vi "Read Stats.vi"(8 "error in (no error)":errorcluster, 11 "System Health Module in":refnum<class "System Health Module.lvclass">) -> (0 "error out":errorcluster, 3 "System Health Module out":refnum<class "System Health Module.lvclass">)   [LabVIEW 2020, in "Volatus.lvlib" / "System Health Module.lvclass"]
uses:
  System Health Module.lvclass
  System Health Module.lvclass/System Health Module.ctl
  System SAL/System SAL.lvclass
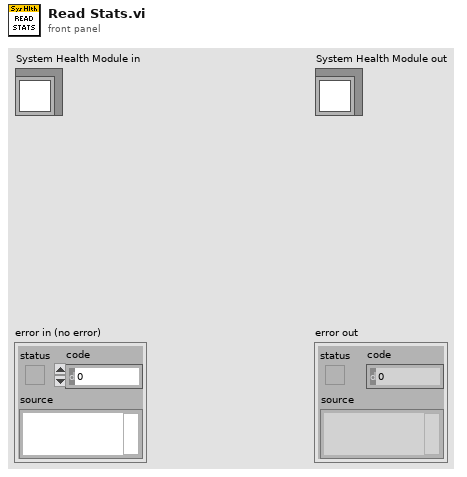
[diagram p1: front panel]
types:
  T1 = typedef "Volatus.lvlib/System Health Module.lvclass/Drive Info.ctl" = cluster{"Config":T2, "Capacity GB":dbl, "Used GB":dbl, "Last Warning":dbl, "Last Error":dbl}
  T2 = typedef "Volatus.lvlib/System Health Module.lvclass/Drive Config.ctl" = cluster{"Path":path, "Warning GB":dbl, "Error GB":dbl}
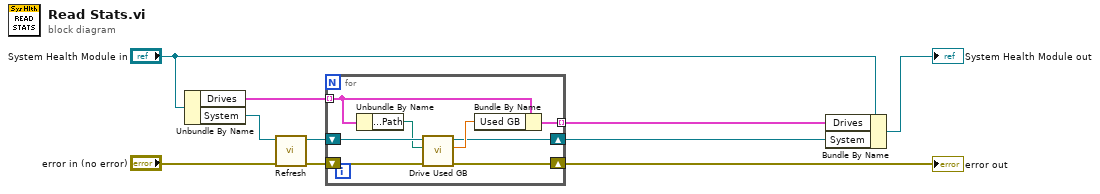
[diagram p0: block diagram]
diagram:
  n1 = Unbundle By Name("System Health Module in") -> ("Drives"=w4:T1[], "System"=w8:refnum<class "System SAL.lvclass">)
  n2 = call-dynamic "Refresh.vi"("error in (no error)"="error in (no error)", "System SAL in"=w8) -> ("error out"=w6:errorcluster, "System SAL out"=w7:refnum<class "System SAL.lvclass">)  [unwired: 8 in]
  n3 = for {
    tunnel: w4 -> [w15] mode=indexing
    shift-right: [w13] -> w2
    shift-left: w7 -> [w18]
    shift-right: [w12] -> w1
    shift-left: w6 -> [w17]
    tunnel: [w11] -> w3 mode=indexing
    n4 = Unbundle By Name(w15) -> ("Config.Path"=w16:path)
    n5 = call-dynamic "Drive Used GB.vi"("error in (no error)"=w17, "Path"=w16, "System SAL in"=w18) -> ("error out"=w12:errorcluster, "Used GB"=w14:dbl, "System SAL out"=w13:refnum<class "System SAL.lvclass">)  [unwired: 6 in]
    n6 = Bundle By Name(cluster=w15, "Used GB"=w14) -> (w11:T1)
  }
  "error out" <- w1
  n7 = Bundle By Name(cluster="System Health Module in", "Drives"=w3, "System"=w2) -> (→"System Health Module out":refnum<class "System Health Module.lvclass">)
